vi "Test_Read_Dataset_With_Start_End.vi"(8 "error in (no error)":errorcluster) -> (0 "error out":errorcluster)   [LabVIEW 2018]
doc: "This VI inits a waveform generation session for AWG-5421. This is a basic example that shows how to setup the board in order to generate waveforms according to a script. \nBy default this configuration uses one channel CH0, and one script trigger ScriptTrigger0. The ScriptTrigger0 is waiting for an external trigger : i.e. a digital Edge on pin PFI 0 by default.\n\nThere are various options for the script to be used. Consult the Script control help for more information on configuring the example for specific scripts."
uses:
  <vilib>/Analysis/NI_AALPro.lvlib
panel:
  in  "End":cluster{i32, i32}(slide) scale=-1.0..3200000.0 scale format="%_1f"
  in  "Cycl. Frequency (kHz)":dbl=255.0 format="%#_13g"
  in  "Start":cluster{i32, i32}(slide) scale=0.0..3200000.0 scale format="%_1f"
  in  "stop":bool
  out "Total Size (bytes) 2":i64
  out "Data Size (samples) 2":i32
  out "Time Step 2":sgl
  out "Vertical Range in data 2":sgl
  out "df 4":dbl caption="df" format="%0.2f"
  out "offset 2":sgl
  out "df 3":dbl caption="df" format="%0.2f"
  out "Mass Spectrum 2":cluster{"mass":sgl[], sgl[]}(graph)
  out "Mass Spectrum":cluster{"mass":sgl[], sgl[]}(graph)
  out "Signal 2":cluster{sgl[], sgl[]}(graph)
  out "Frequency Spectrum 2":cluster{dbl[], "Power Spectrum (V^2 rms)":dbl[]}(graph)
  out "Frequency Spectrum":cluster{dbl[], "Power Spectrum (V^2 rms)":dbl[]}(graph)
  out "Signal":cluster{sgl[], sgl[]}(graph)
  in  "chemin du fichier":path=path "D:/PIRENEA/DATA/2017/data_2017_06_09/2017_06_09_003.A00"
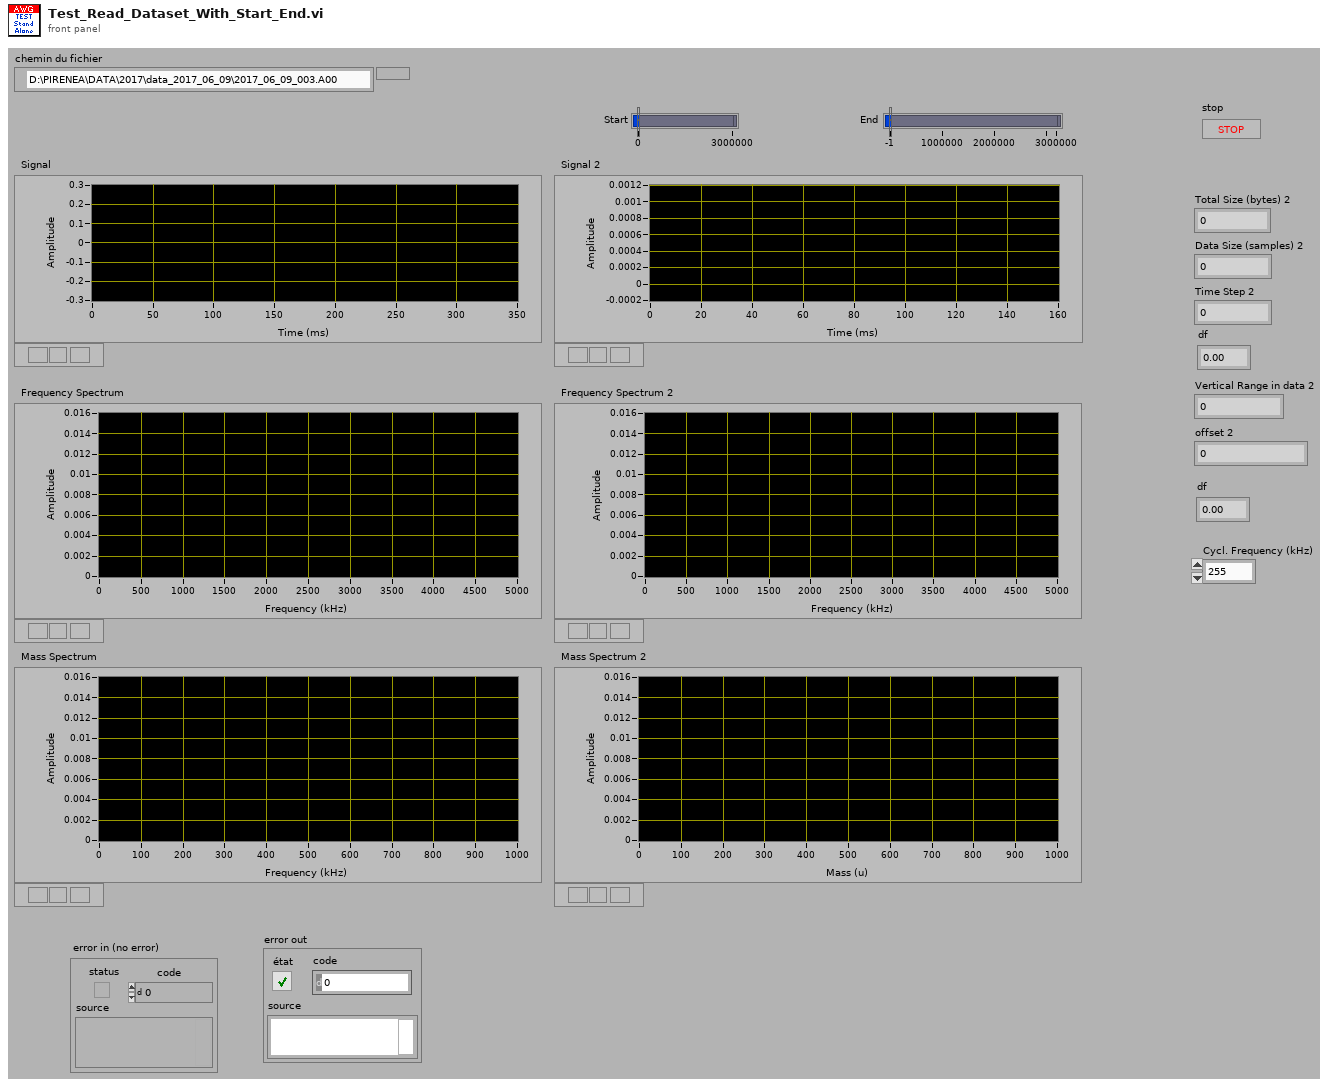
[diagram p1: front panel]
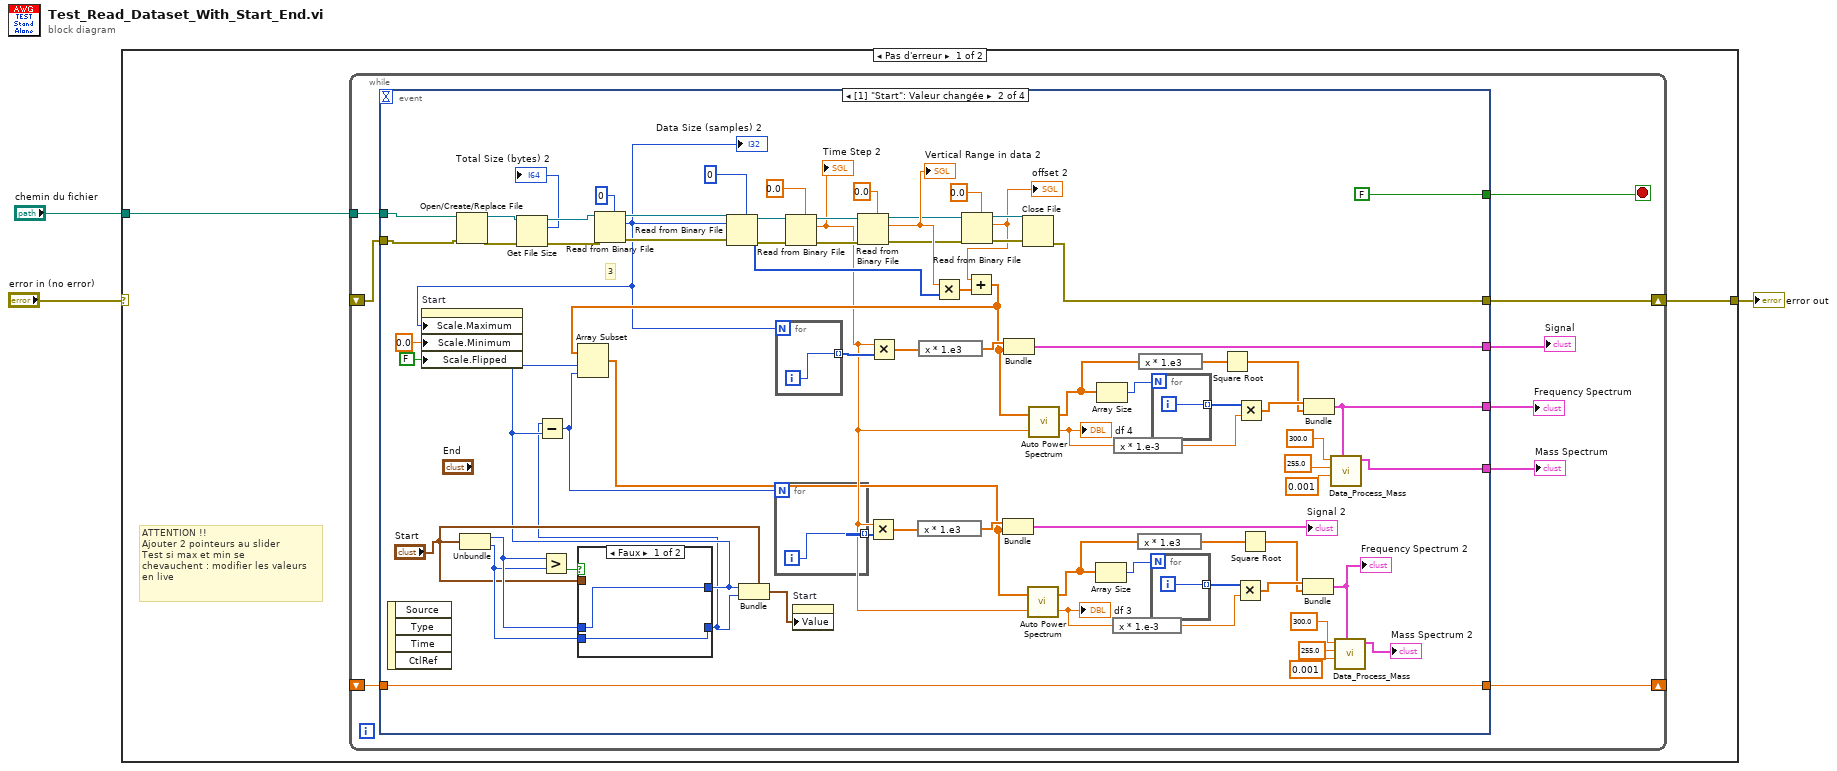
[diagram p0: block diagram]
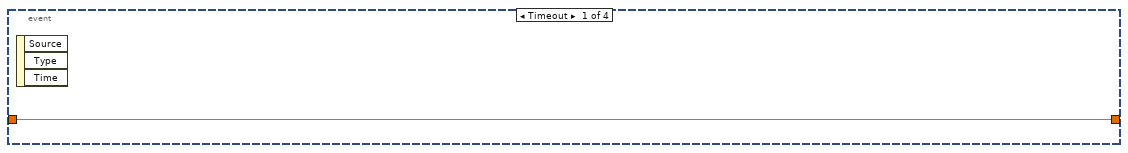
[diagram p2: hidden frame]
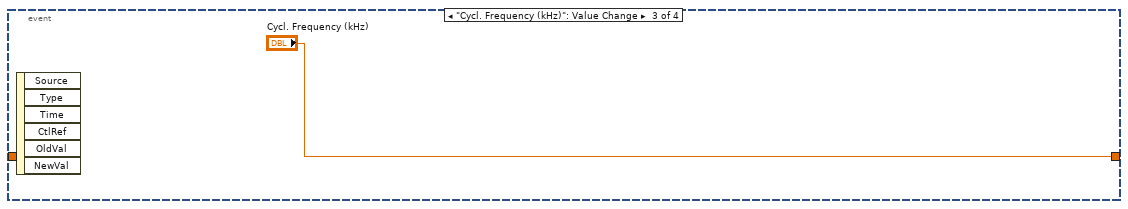
[diagram p4: hidden frame]
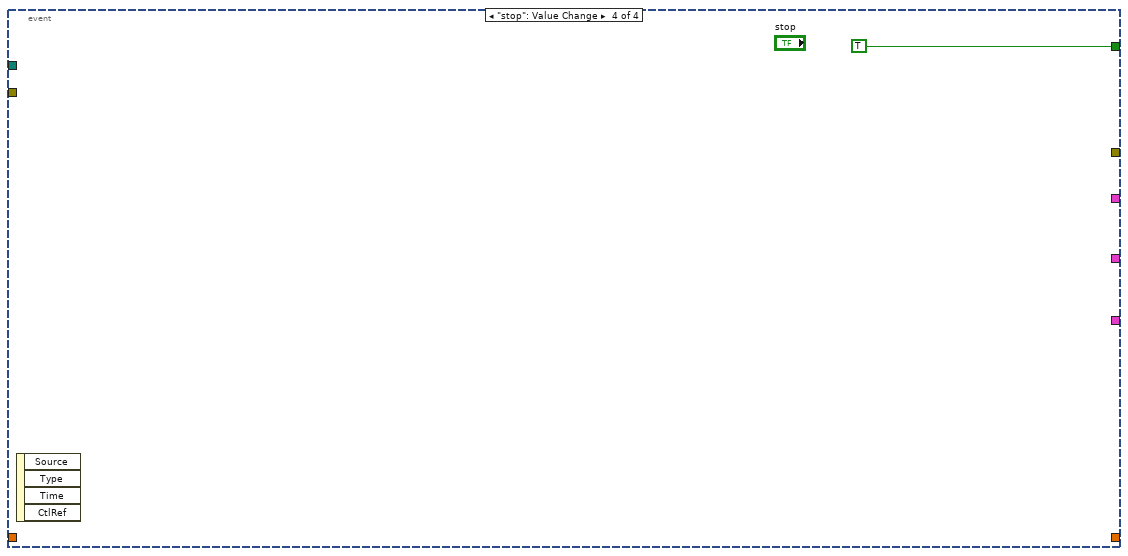
[diagram p5: hidden frame]
diagram:
  n1 = case shown="Pas d'erreur" "error in (no error)" {
    selector: "error in (no error)" -> [_ w103]
    tunnel: [w4 w103] -> w3
    tunnel: "chemin du fichier" -> [w5 _]
    frame No Error {
      # "ATTENTION !!\nAjouter 2 pointeurs au slider\nTest si max et min se\nchevauchent : modifier les valeurs\nen live"
      n2 = while {
        tunnel: w5 -> [w14]
        shift-right: [w13] -> w4
        shift-left: _ -> [w12]
        shift-right: [w7] -> _
        shift-left: _ -> [w8]
        stop <- w11 stop-if-true
        n3 = event shown="[1] \"Start\": Valeur changée" {
          selector: _ -> [_ _ _ _]
          dyn-events: _ -> [_ _ _ _]
          timeout: _ -> [_ _ _ _]
          tunnel: w14 -> [_ w83 _ _]
          tunnel: [_ w76 _ _] -> w13
          tunnel: [_ w41 _ _] -> w10
          tunnel: w12 -> [_ w32 _ _]
          tunnel: [_ FALSE _ TRUE] -> w11
          tunnel: [_ w27 _ _] -> w9
          tunnel: w8 -> [w15 w26 _ _]
          tunnel: [w15 w26 "Cycl. Frequency (kHz)" _] -> w7
          tunnel: [_ w25 _ _] -> w6
          event Timeout {
            n4 = event-data() -> ()  [unwired: 1 in, 3 out]
          }
          event "Start": Value Change {
            # "3"
            n5 = event-data() -> ()  [unwired: 1 in, 4 out]
            n6 = Open/Create/Replace File(file path (use dialog)=w83, error in=w32) -> (refnum out=w91:refnum<file>, error out=w90:errorcluster)  [unwired: 4 in, 1 out]
            n7 = Unbundle("Start") -> (w36:i32, w35:i32)
            n8 = Get File Size(file=w91, error in=w90) -> (refnum out=w89:refnum<file>, size (in bytes)=→"Total Size (bytes) 2":i64, 0:w88:errorcluster)
            n9 = Greater?(x=w36, y=w35) -> (0:w39:bool)
            n10 = case shown="Faux" w39 {
              tunnel: "Start" -> [_ _]
              tunnel: w36 -> [w94 w95]
              tunnel: w35 -> [w93 w96]
              tunnel: [w94 w96] -> w31
              tunnel: [w93 w95] -> w30
              frame False {
              }
              frame True {
              }
            }
            n11 = Subtract(x=w30, y=w31) -> (x-y=w46:i32)
            n12 = Read from Binary File(5:0, 8:w88, 11:w89) -> (0:w85:errorcluster, 2:w29:i32, 3:w86:refnum<file>)  [unwired: 3 in, 1 out]
            "Data Size (samples) 2" <- w29
            n13 = property on="Start" class="Gliss (strict)"("Scale.Maximum"=w29, "Scale.Minimum"=0.0 ("Échelle.Gamme:Minimum"), "Scale.Flipped"=FALSE ("Échelle.Inversée")) -> ()  [unwired: 2 in, 2 out]
            n14 = Read from Binary File(5:i16 0, 8:w85, 10:w29, 11:w86) -> (0:w81:errorcluster, 2:w75:i16[], 3:w82:refnum<file>)  [unwired: 2 in, 1 out]
            n15 = Bundle(cluster="Start", w31, w30) -> (w28:cluster{i32, i32})
            n16 = for {
              N: w46 -> [_]
              tunnel: [w100] -> w47 mode=indexing
              i -> [w100]
            }
            n17 = for {
              N: w29 -> [_]
              tunnel: [w98] -> w74 mode=indexing
              i -> [w98]
            }
            n18 = Read from Binary File(5:sgl 0.0 ("type de données"), 8:w81, 11:w82) -> (0:w79:errorcluster, 2:w45:sgl, 3:w78:refnum<file>)  [unwired: 3 in, 1 out]
            "Time Step 2" <- w45
            n19 = property on="Start" class="Gliss (strict)"("Value"=w28) -> ()  [unwired: 2 in, 2 out]
            n20 = Read from Binary File(5:sgl 0.0 ("type de données"), 8:w79, 11:w78) -> (0:w70:errorcluster, 2:w73:sgl, 3:w72:refnum<file>)  [unwired: 3 in, 1 out]
            "Vertical Range in data 2" <- w73
            n21 = Multiply(x=w45, y=w47) -> (x*y=w53:sgl[])
            n22 = Multiply(x=w45, y=w74) -> (x*y=w60:sgl[])
            n23 = expression code="x * 1.e3"(w53) -> (w54:sgl[])
            n24 = expression code="x * 1.e3"(w60) -> (w59:sgl[])
            n25 = Multiply(x=w73, y=w75) -> (x*y=w67:sgl[])
            n26 = Read from Binary File(5:sgl 0.0, 8:w70, 11:w72) -> (0:w69:errorcluster, 2:w66:sgl, 3:w71:refnum<file>)  [unwired: 3 in, 1 out]
            "offset 2" <- w66
            n27 = Add(x=w66, y=w67) -> (x+y=w56:sgl[])
            n28 = Array Subset(array=w56, index=w31, length=w46) -> (w44:sgl[])
            n29 = Bundle(w54, w44) -> (→"Signal 2":cluster{sgl[], sgl[]})  [unwired: 1 in]
            n30 = Bundle(w59, w56) -> (w27:cluster{sgl[], sgl[]})  [unwired: 1 in]
            n31 = Close File(refnum=w71, error in=w69) -> (error out=w76:errorcluster)  [unwired: 1 out]
            n32 = call <vilib>:"Auto Power Spectrum.vi"("dt"=w45, "Signal (V)"=w44) -> ("df"=w51:dbl, "Power Spectrum (V^2 rms)"=w55:dbl[])
            "df 3" <- w51
            n33 = call <vilib>:"Auto Power Spectrum.vi"("dt"=w45, "Signal (V)"=w56) -> ("df"=w62:dbl, "Power Spectrum (V^2 rms)"=w58:dbl[])
            "df 4" <- w62
            n34 = Array Size(array=w55) -> (size(s)=w48:i32)
            n35 = Array Size(array=w58) -> (size(s)=w65:i32)
            n36 = expression code="x * 1.e-3"(w51) -> (w52:dbl)
            n37 = expression code="x * 1.e-3"(w62) -> (w61:dbl)
            n38 = expression code="x * 1.e3"(w55) -> (w43:dbl[])
            n39 = expression code="x * 1.e3"(w58) -> (w57:dbl[])
            n40 = for {
              N: w48 -> [_]
              tunnel: [w99] -> w49 mode=indexing
              i -> [w99]
            }
            n41 = for {
              N: w65 -> [_]
              tunnel: [w97] -> w64 mode=indexing
              i -> [w97]
            }
            n42 = Square Root(x=w57) -> (sqrt(x)=w40:dbl[])
            n43 = Multiply(x=w49, y=w52) -> (x*y=w50:dbl[])
            n44 = Multiply(x=w64, y=w61) -> (x*y=w63:dbl[])
            n45 = Square Root(x=w43) -> (sqrt(x)=w42:dbl[])
            n46 = Bundle(w50, w42) -> (w34:cluster{dbl[], dbl[]})  [unwired: 1 in]
            "Frequency Spectrum 2" <- w34
            n47 = Bundle(w63, w40) -> (w41:cluster{dbl[], dbl[]})  [unwired: 1 in]
            n48 = call "Data_Process_Mass.vi"("Frequency Spectrum"=w41, "Mag. Frequency (kHz)"=0.001, "Cycl. Frequency (kHz)"=255.0, "Reference mass (u)"=300.0) -> ("Mass Spectrum"=w25:cluster{"mass":sgl[], sgl[]})  [unwired: 6 in, 1 out]
            n49 = call "Data_Process_Mass.vi"("Frequency Spectrum"=w34, "Mag. Frequency (kHz)"=0.001, "Cycl. Frequency (kHz)"=255.0, "Reference mass (u)"=300.0) -> ("Mass Spectrum"=→"Mass Spectrum 2":cluster{"mass":sgl[], sgl[]})  [unwired: 6 in, 1 out]
          }
          event "Cycl. Frequency (kHz)": Value Change {
            n50 = event-data() -> ()  [unwired: 1 in, 6 out]
          }
          event "stop": Value Change {
            n51 = event-data() -> ()  [unwired: 1 in, 4 out]
          }
        }
        "Frequency Spectrum" <- w10
        "Mass Spectrum" <- w6
        "Signal" <- w9
      }
    }
    frame Error {
    }
  }
  "error out" <- w3
